vi "Map Tags to Channels.vi"(7 "instance id":string, 8 "error in (no error)":errorcluster, 9 "String Array":string[][](array[string]), 10 "tag select":T1[](array[typedef]), 11 "engine in":refnum<class "engine configuration.lvclass">) -> (0 "error out":errorcluster, 3 "engine out":refnum<class "engine configuration.lvclass">)   [LabVIEW 2015, in "tag select module editor node.lvclass"]
uses:
  tag select module editor node.lvclass
  <vilib>/NI/Module Execution Interface/Engine Configuration/engine configuration.lvclass
  module/configuration/tag select configuration.ctl
  <vilib>/NI/Tag Bus Module Framework/channel/TBM channel.lvclass
  <vilib>/NI/Tag Bus/tag/Data Type.ctl
  <vilib>/NI/Tag Bus/tag/tag descriptor.lvclass/tag descriptor.ctl
  <vilib>/NI/Tag Bus/tag/tag descriptor.lvclass
  module/configuration/tag select module configuration.lvclass
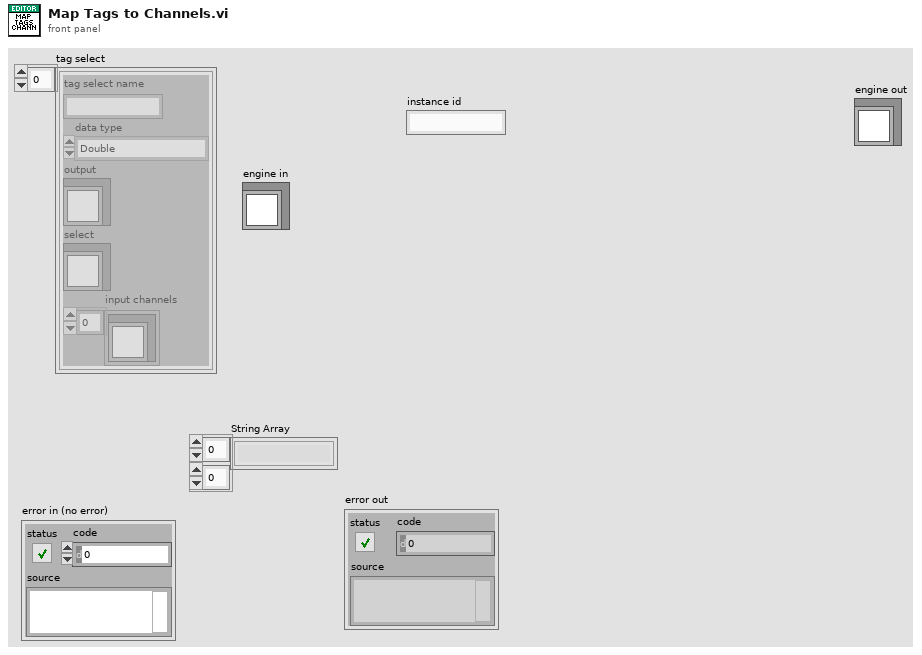
[diagram p1: front panel]
types:
  T1 = typedef "tag select module configuration.lvclass/tag select configuration.ctl" = cluster{"tag select name":string, "data type":T2, "output":refnum<class "TBM channel.lvclass">, "select":refnum<class "TBM channel.lvclass">, "input channels":refnum<class "TBM channel.lvclass">[]}
  T2 = typedef "tag bus.lvlib/tag descriptor.lvclass/Data Type.ctl" = enum16{"Double", "Single", "I64", "I32", "I16", "I8", "U64", "U32", "U16", "U8", "Boolean", "String", "Array of Double", "Array of Single", "Array of I64", "Array of I32", "Array of I16", "Array of I8", "Array of U64", "Array of U32", "Array of U16", "Array of U8", "Array of Boolean", "Array of String"}
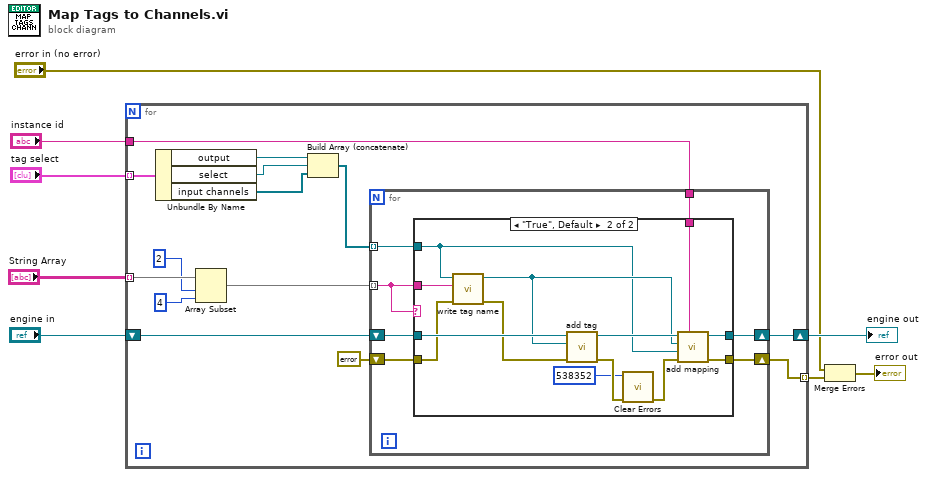
[diagram p0: block diagram]
diagram:
  n1 = for {
    shift-right: [w18] -> w7
    shift-left: "engine in" -> [w21]
    tunnel: "tag select" -> [w22] mode=indexing
    tunnel: "String Array" -> [w12] mode=indexing
    tunnel: "instance id" -> [w20]
    tunnel: [w19] -> w1 mode=indexing
    n2 = Unbundle By Name(w22) -> ("output"=w17:refnum<class "TBM channel.lvclass">, "select"=w16:refnum<class "TBM channel.lvclass">, "input channels"=w15:refnum<class "TBM channel.lvclass">[])
    n3 = Array Subset "Array Subset"(array=w12, index=2, length=4) -> (w9:string[])
    n4 = Build Array (concatenate)(w17, w16, w15) -> (w14:refnum<class "TBM channel.lvclass">[])
    n5 = for {
      shift-right: [w28] -> w18
      shift-left: w21 -> [w29]
      tunnel: w20 -> [w27]
      shift-right: [w26] -> w19
      shift-left: errorcluster {"status"=FALSE, "code"=0, "source"=""} ("error out") -> [w25]
      tunnel: w14 -> [w24] mode=indexing
      tunnel: w9 -> [w23] mode=indexing
      n6 = case shown="\"True\", Default" w23 {
        tunnel: w29 -> [w31 w40]
        tunnel: [w31 w39] -> w28
        tunnel: w27 -> [_ w38]
        tunnel: [w30 w37] -> w26
        tunnel: w23 -> [_ w36]
        tunnel: w25 -> [w30 w35]
        tunnel: w24 -> [_ w32]
        frame "\u0000" {
        }
        frame "True", Default {
          n7 = call <vilib>:"write tag name.vi"("error in"=w35, "name"=w36, "system tag in"=w32) -> ("error out"=w34:errorcluster, "system tag out"=w33:refnum<class "TBM channel.lvclass">)  [unwired: 7 in]
          n8 = call-dynamic "add tag.vi"("error in"=w34, "tag descriptor"=w33, "engine configuration in"=w40) -> ("error out"=w43:errorcluster, "engine configuration out"=w44:refnum<class "engine configuration.lvclass">)  [unwired: 7 in]
          n9 = call <vilib>:"Clear Errors.vi"("error in (no error)"=w43, "specific error code to clear (0: all)"=538352) -> ("error out"=w42:errorcluster)  [unwired: 4 in, 1 out]
          n10 = call-dynamic "add mapping.vi"("owner ID"=w38, "error in"=w42, "channel"=w32, "tag descriptor"=w33, "engine configuration"=w44) -> ("error out"=w37:errorcluster, "engine configuration out"=w39:refnum<class "engine configuration.lvclass">)  [unwired: 5 in]
        }
      }
    }
  }
  "engine out" <- w7
  n11 = Merge Errors("error in (no error)", w1) -> (→"error out":errorcluster)
